vi "Drop Stack.vi"(8 "error in":errorcluster, 11 "Auto Notifiers In":T1) -> (0 "error out":errorcluster, 3 "Auto Notifiers Out":T1)   [LabVIEW 2014]
doc: "Sets elevator to Ground"
uses:
  Auto Notifiers.ctl
  Main/Arms/Arm clapper state.ctl
  Main/Arms/Arm State.ctl
  Main/Elevator/Elevator States.ctl
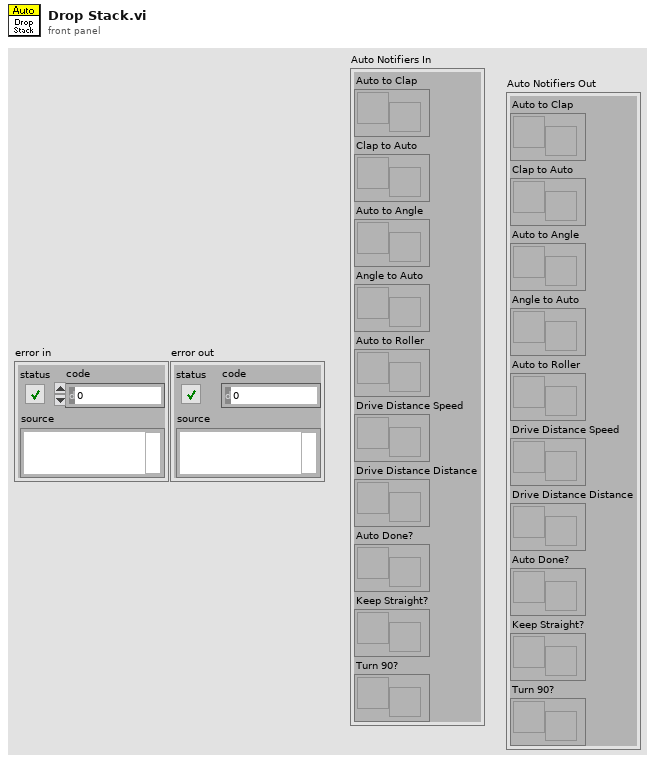
[diagram p1: front panel]
types:
  T1 = typedef "Auto Notifiers.ctl" = cluster{"Auto to Clap":refnum<notifier>, "Clap to Auto":refnum<notifier>, "Auto to Angle":refnum<notifier>, "Angle to Auto":refnum<notifier>, "Auto to Roller":refnum<notifier>, "Drive Distance Speed":refnum<notifier>, "Drive Distance Distance":refnum<notifier>, "Auto Done?":refnum<notifier>, "Keep Straight?":refnum<notifier>, "Turn 90?":refnum<notifier>}
  T2 = typedef "Elevator States.ctl" = enum16{"Ground", "Tote 1", "Tote 2", "Tote 3", "Tote 4", "Tote 5", "Tote 6"}
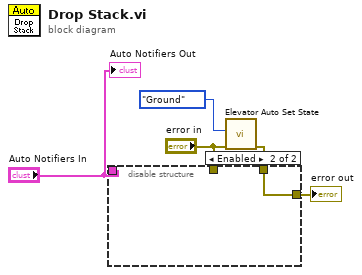
[diagram p0: block diagram]
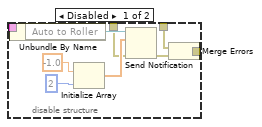
[diagram p2: hidden frame]
diagram:
  n1 = call "Elevator Auto Set State.vi"("error in (no error)"="error in", "New State"=Elevator_States."Ground" ("Auto Input State")) -> ("error out"=w2:errorcluster)  [unwired: 9 in]
  n2 = disable-structure shown="Enabled" {
    disable-tunnel: "Auto Notifiers In" -> [w14 _]
    disable-tunnel: [w9 w15] -> w3
    disable-tunnel: w2 -> [w8 w15]
    disable-tunnel: "error in" -> [w7 _]
    frame Disabled {
      n3 = Unbundle By Name(w14) -> ("Auto to Roller"=w13:refnum<notifier>)
      n4 = Initialize Array(-1.0 ("element"), 2 ("dimension size")) -> (w10:dbl[])
      n5 = Send Notification(notification=w10, notifier=w13, error in (no error)=w7) -> (error out=w6:errorcluster)  [unwired: 1 out]
      n6 = Merge Errors(w8, w6) -> (w9:errorcluster)
    }
    frame Enabled {
    }
  }
  "error out" <- w3
  "Auto Notifiers Out" <- "Auto Notifiers In"
